vi "Set Message class icon.vi"() -> ()   [LabVIEW 2015]
panel:
  in  "Project Path":path
  in  "My Computer?":bool
  in  "Array":path[](array[path])
  in  "Path":path
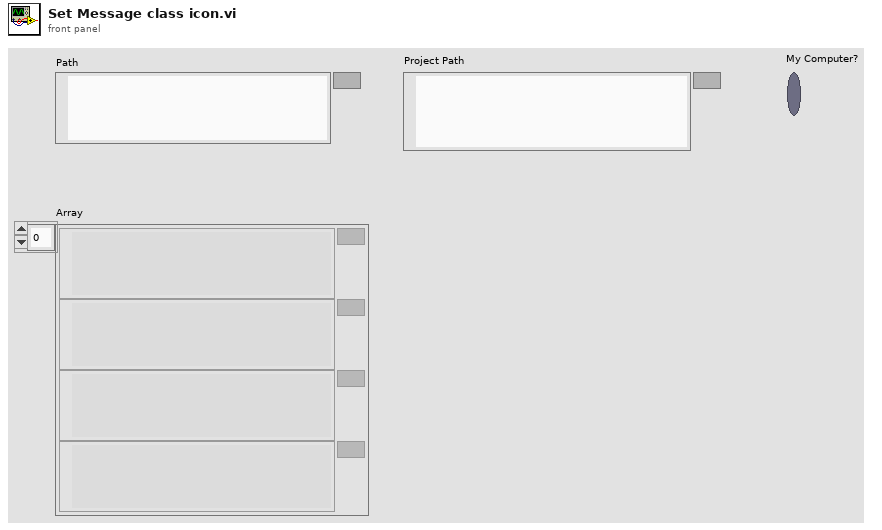
[diagram p1: front panel]
types:
  T1 = typedef "imagedata.ctl" = cluster{"image type":i32, "image depth":i32, "image":u8[], "mask":u8[], "colors":u32[], "Rectangle":cluster{"left":i16, "top":i16, "right":i16, "bottom":i16}}
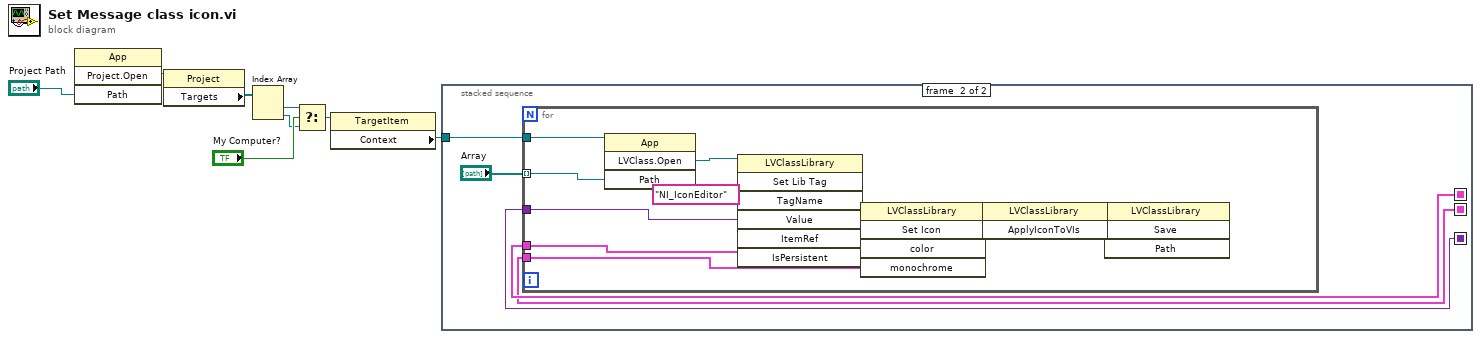
[diagram p0: block diagram]
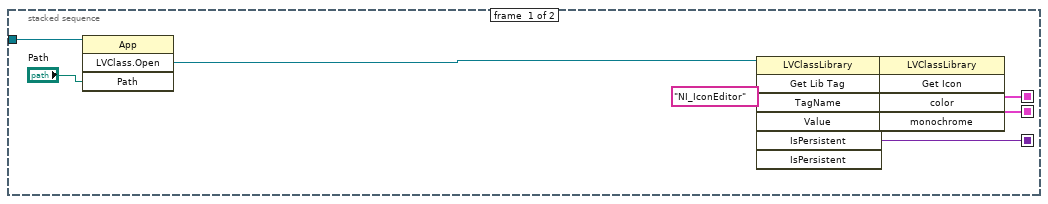
[diagram p2: hidden frame]
diagram:
  n1 = invoke class="App" method="Project.Open"("Path"="Project Path") -> ("Project:Open"=w8:refnum<vi>)  [unwired: 3 in, 3 out]
  n2 = property class="Project"(reference=w8) -> ("Targets"=w7:refnum<vi>[])  [unwired: 1 in, 2 out]
  n3 = Index Array(array=w7) -> (element #1=w4:refnum<vi>, element #2=w3:refnum<vi>)  [unwired: 2 in]
  n4 = Select(t=w4, s="My Computer?", f=w3) -> (s? t:f=w2:refnum<vi>)
  n5 = property class="TargetItem"(reference=w2) -> ("Context"=w1:refnum<vi>)  [unwired: 1 in, 2 out]
  n6 = stacked-sequence {
    seq-local: [w11 _] -> [_ w19]
    seq-local: [w10 _] -> [_ w18]
    seq-local: [w9 _] -> [_ w17]
    tunnel: w1 -> [w12 w20]
    frame #0 {
      n7 = invoke class="App" method="LVClass.Open"(reference=w12, "Path"="Path") -> ("LVClass.Open"=w13:refnum<vi>)  [unwired: 2 in, 3 out]
      n8 = invoke class="LVClassLibrary" method="Get Lib Tag"(reference=w13, "TagName"="NI_IconEditor" ("Tag Name")) -> (reference out=w16:refnum<vi>, "Value"=w11:variant)  [unwired: 5 in, 5 out]
      n9 = invoke class="LVClassLibrary" method="Get Icon"(reference=w16) -> ("color"=w10:T1, "monochrome"=w9:T1)  [unwired: 4 in, 3 out]
    }
    frame #1 {
      n10 = for {
        tunnel: "Array" -> [w27] mode=indexing
        tunnel: w18 -> [w25]
        tunnel: w17 -> [w24]
        tunnel: w19 -> [w23]
        tunnel: w20 -> [w22]
        n11 = invoke class="App" method="LVClass.Open"(reference=w22, "Path"=w27) -> ("LVClass.Open"=w28:refnum<vi>)  [unwired: 2 in, 3 out]
        n12 = invoke class="LVClassLibrary" method="Set Lib Tag"(reference=w28, "TagName"="NI_IconEditor" ("Tag Name"), "Value"=w23) -> (reference out=w29:refnum<vi>)  [unwired: 4 in, 6 out]
        n13 = invoke class="LVClassLibrary" method="Set Icon"(reference=w29, "color"=w25, "monochrome"=w24) -> (reference out=w30:refnum<vi>)  [unwired: 2 in, 4 out]
        n14 = invoke class="LVClassLibrary" method="ApplyIconToVIs"(reference=w30) -> (reference out=w31:refnum<vi>)  [unwired: 2 in, 2 out]
        n15 = invoke class="LVClassLibrary" method="Save"(reference=w31) -> ()  [unwired: 3 in, 4 out]
      }
    }
  }
